vi "Get LR700 data.vi"   [LabVIEW 2015]
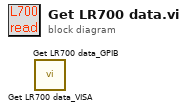
[diagram p0: block diagram]
diagram:
  n1 = call "Get LR700 data_VISA.vi"() -> ()  [unwired: 5 in, 3 out]
  n2 = call "Get LR700 data_GPIB.vi"() -> ()  [unwired: 6 in, 2 out]
